vi "Load_Array_Data_to_File_txt.vi"(6 "format string(%.5f)":string="%.5f", 7 "delimiter (comma)":string=",", 8 "error in":errorcluster, 9 "array type":string[][](array[string]), 11 "file path (use dialog)":path) -> (0 "error out":errorcluster, 2 "text(raw)":string, 3 "array":string[][](array[string]))   [LabVIEW 2015]
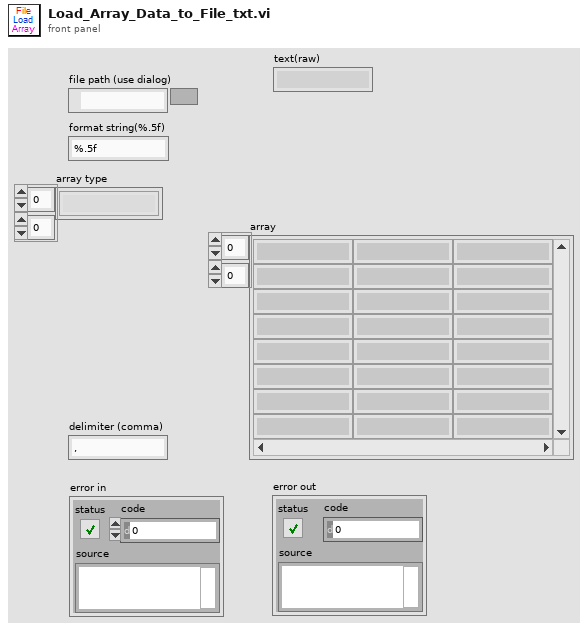
[diagram p1: front panel]
types:
  T1 = enum16{"open", "replace", "create", "open or create", "replace or create", "replace or create with confirmation"}
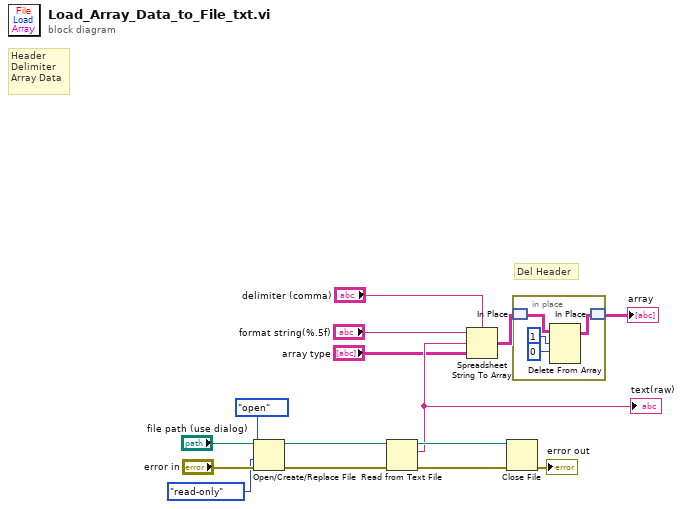
[diagram p0: block diagram]
diagram:
  # "Del Header"
  # "Header\nDelimiter\nArray Data"
  n1 = Open/Create/Replace File(file path (use dialog)="file path (use dialog)", error in="error in", operation (0:open)=T1."open", access (0:read/write)=enum16{"read/write", "read-only", "write-only"}."read-only") -> (refnum out=w15:refnum<file>, error out=w14:errorcluster)  [unwired: 2 in, 1 out]
  n2 = Read from Text File(file (use dialog)=w15, error in=w14) -> (refnum out=w13:refnum<file>, text=w6:string, error out=w12:errorcluster)  [unwired: 2 in, 1 out]
  "text(raw)" <- w6
  n3 = Spreadsheet String To Array(delimiter (Tab)="delimiter (comma)", format string="format string(%.5f)", spreadsheet string=w6, array type (2D Dbl)="array type") -> (array=w3:string[][])
  n4 = Close File(refnum=w13, error in=w12) -> (error out=→"error out":errorcluster)  [unwired: 1 out]
  n5 = in-place {
    n6 = in-place-match #1(w3) -> (w19:string[][])
    n7 = Delete From Array(array=w19, length=1, index (row)=0) -> (array with subset deleted=w16:string[][])  [unwired: 1 in, 1 out]
    n8 = in-place-match #1(w16) -> (→"array":string[][])
  }
